vi "Modal Sub-VI.vi"(8 "error in (no error)":errorcluster) -> (0 "error out":errorcluster)   [LabVIEW 2026]
panel:
  out "File Name 1":string caption="File Name"
  in  "Frame Sync Edge for Channel 0":enum16{"Rising", "Falling"}(ring)=enum."Falling"
  in  "Endianness":enum16{"MSB First", "LSB First"}(ring)
  in  "Data Justification":enum16{"Left Justified", "Right Justified"}(ring)
  in  "Channel Count Per Frame":i32=2
  in  "Channel Length":i32=32
  in  "Bit Depth":i32=24
  in  "Channel 0 Offset":i32=1
  in  "Frame Length":i32=64
  in  "Frame Sync Pulse Width":i32=32
  in  "Bit Clock Edge  Sync":enum16{"Rising", "Falling"}(ring)=enum."Falling"
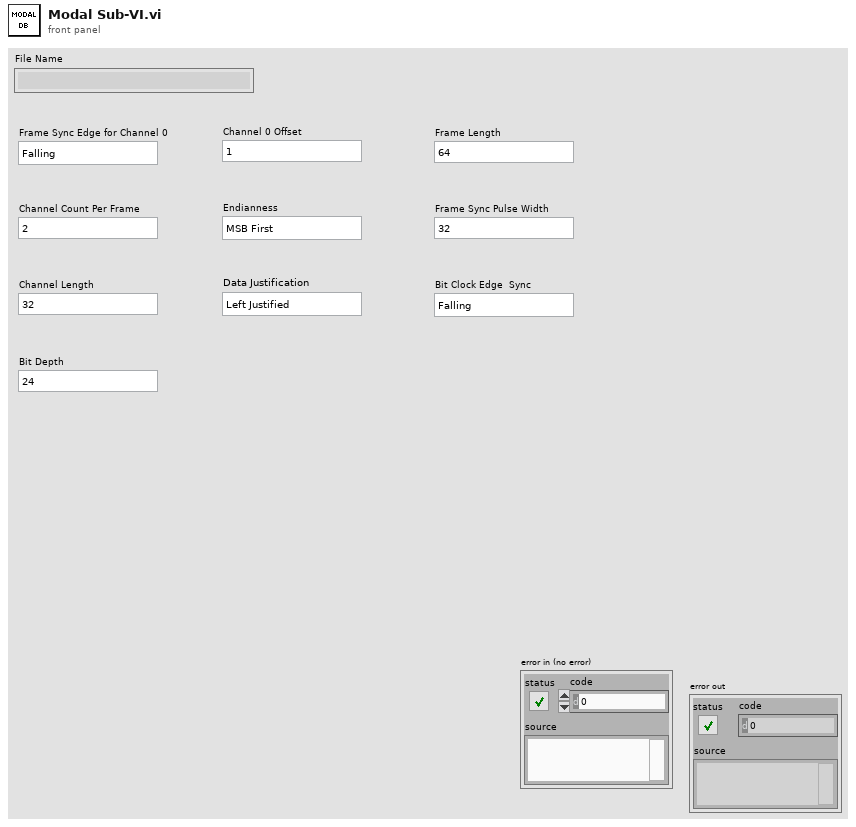
[diagram p1: front panel]
types:
  T1 = enum32{"Invalid", "Standard", "Closed", "Hidden", "Minimized", "Maximized"}
  T2 = cluster{"Configurations":cluster{"Frame_Sync_Edge_for_Channel 0":i32, "Channel_Count_Per_Frame":i32, "Channel_Length":i32, "Bit_Depth":i32, "Channel_0_Offset":i32, "Endianness":i32, "Data_Justification":i32, "Frame_Length":i32, "Frame_Sync_Pulse_Width":i32, "Bit_Clock_Edge_Sync":i32}}
  T3 = enum16{"open", "replace", "create", "open or create", "replace or create", "replace or create with confirmation"}
  T4 = cluster{"Frame_Sync_Edge_for_Channel 0":i32, "Channel_Count_Per_Frame":i32, "Channel_Length":i32, "Bit_Depth":i32, "Channel_0_Offset":i32, "Endianness":i32, "Data_Justification":i32, "Frame_Length":i32, "Frame_Sync_Pulse_Width":i32, "Bit_Clock_Edge_Sync":i32}
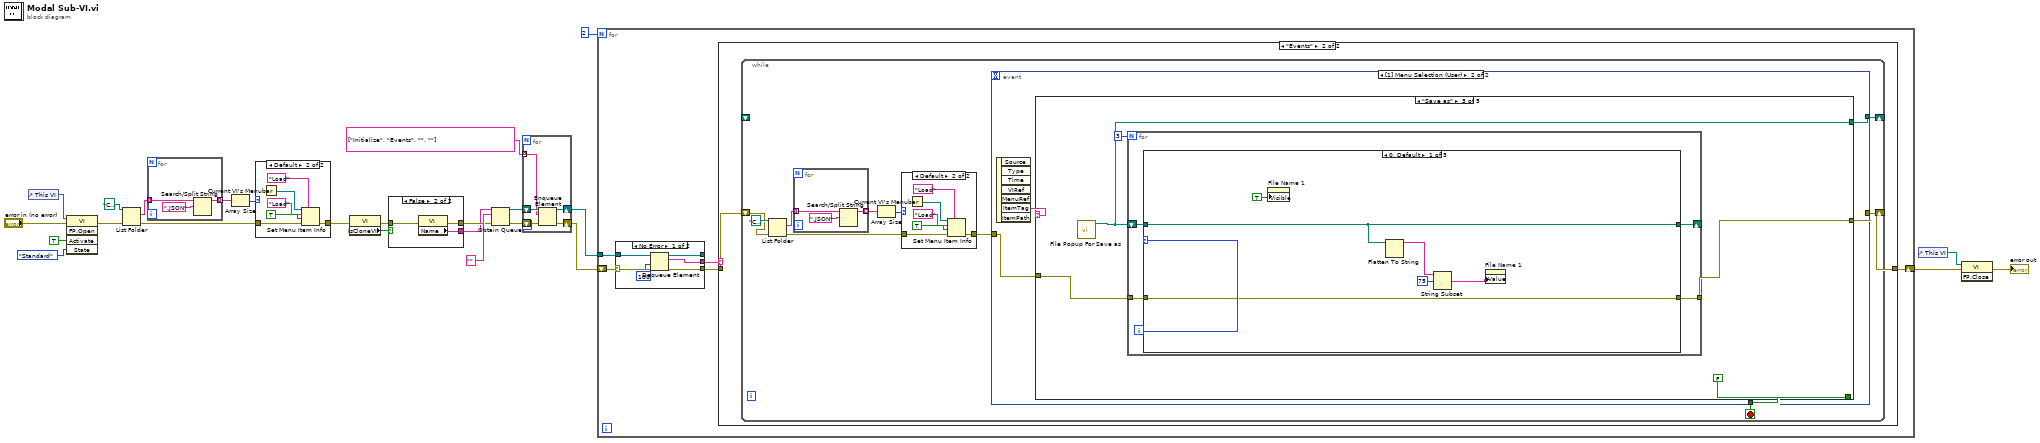
[diagram p0: block diagram]
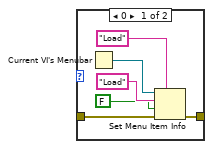
[diagram p2: hidden frame]
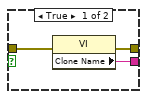
[diagram p3: hidden frame]
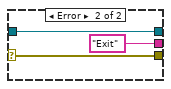
[diagram p4: hidden frame]
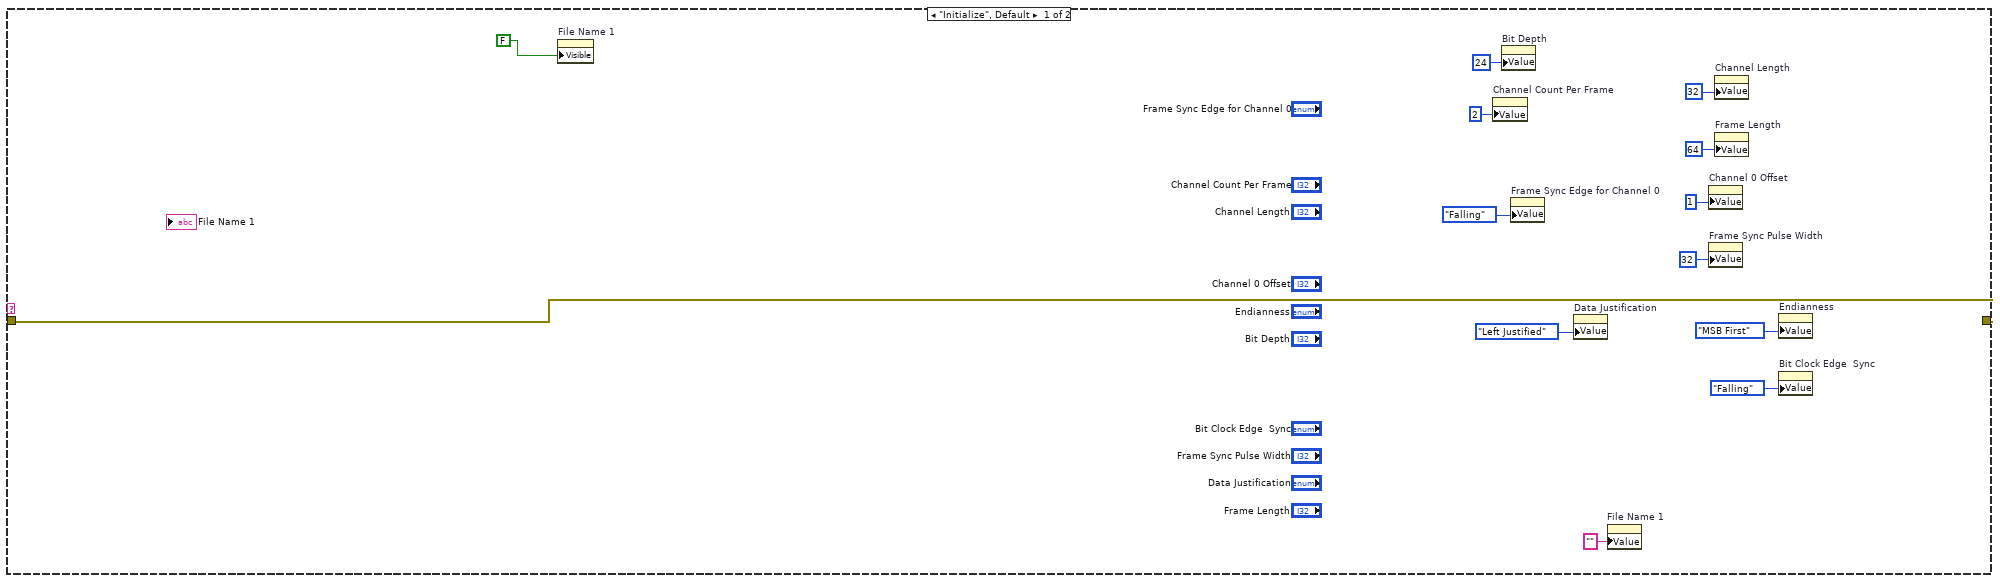
[diagram p5: hidden frame]
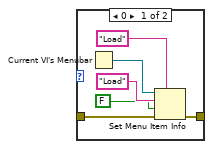
[diagram p6: hidden frame]
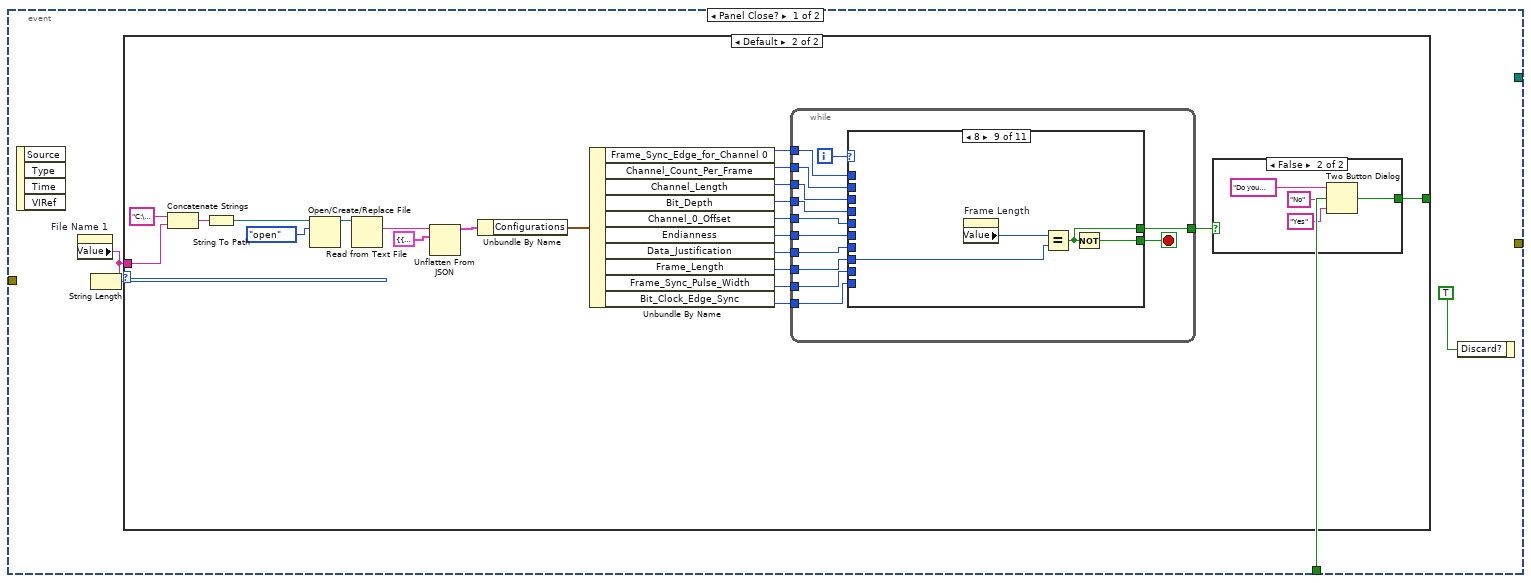
[diagram p7: hidden frame]
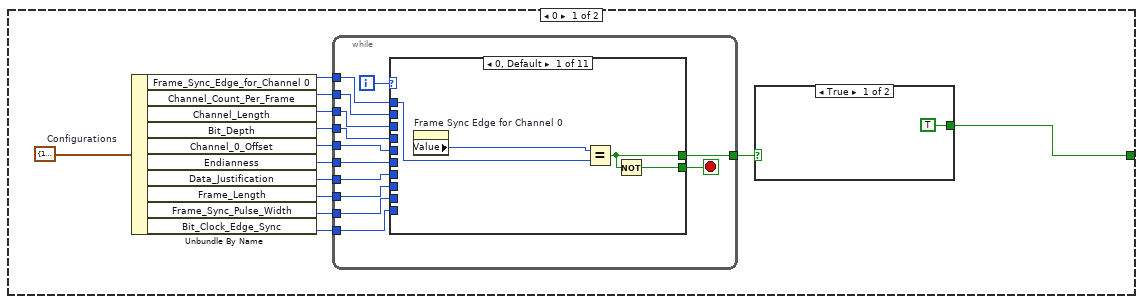
[diagram p8: hidden frame]
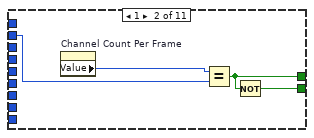
[diagram p9: hidden frame]
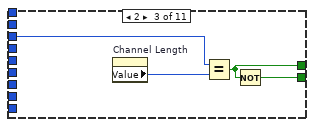
[diagram p10: hidden frame]
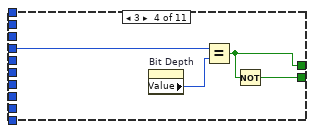
[diagram p11: hidden frame]
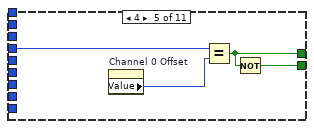
[diagram p12: hidden frame]
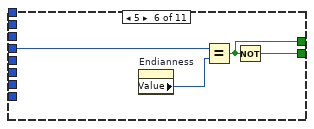
[diagram p13: hidden frame]
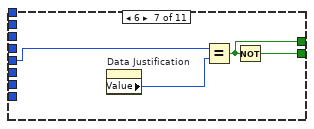
[diagram p14: hidden frame]
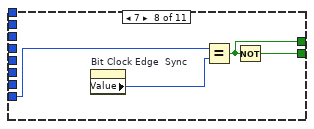
[diagram p15: hidden frame]
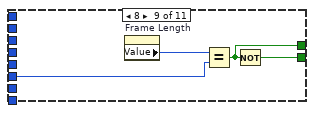
[diagram p16: hidden frame]
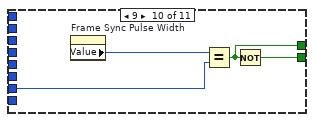
[diagram p17: hidden frame]
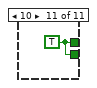
[diagram p18: hidden frame]
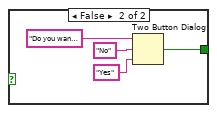
[diagram p19: hidden frame]
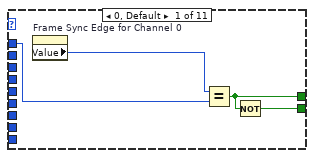
[diagram p20: hidden frame]
diagram:
  n1 = control-ref of="This VI"() -> (w25:refnum<vi>)
  n2 = invoke class="VI" method="FP.Open"(reference=w25, error in="error in (no error)", "Activate"=TRUE ("Activate?"), "State"=T1."Standard") -> (error out=w2:errorcluster)  [unwired: 1 in, 4 out]
  n3 = List Folder(path=path "C:/Users/Public/Documents/National Instruments/Audio/Protocols", error in=w2) -> (filenames=w3:string[], error out=w7:errorcluster)  [unwired: 2 in, 2 out]
  n4 = for {
    tunnel: w3 -> [w27] mode=indexing
    tunnel: [w26] -> w5 mode=indexing
    n5 = Search/Split String(string=w27, search string/char (-)=".JSON") -> (substring before match=w26:string)  [unwired: 1 in, 2 out]
  }
  n6 = Array Size(array=w5) -> (size(s)=w6:i32)
  n7 = case shown="Default" w6 {
    tunnel: w7 -> [w31 w38]
    tunnel: [w30 w37] -> w1
    frame 0 {
      n8 = Current VI's Menubar() -> (w34:refnum<k9>)
      n9 = Set Menu Item Info(7:"Load" ("item tag"), 8:w31, 9:FALSE ("enabled"), 10:"Load" ("item name"), 11:w34) -> (0:w30:errorcluster)  [unwired: 2 in, 1 out]
    }
    frame Default {
      n10 = Current VI's Menubar() -> (w35:refnum<k9>)
      n11 = Set Menu Item Info(7:"Load" ("item tag"), 8:w38, 9:TRUE ("enabled"), 10:"Load" ("item name"), 11:w35) -> (0:w37:errorcluster)  [unwired: 2 in, 1 out]
    }
  }
  n12 = property class="VI"(error in=w1) -> (error out=w14:errorcluster, "IsCloneVI"=w15:bool)  [unwired: 1 in, 1 out]
  n13 = case shown="False" w15 {
    tunnel: [w43 w46] -> w13
    tunnel: [w42 w45] -> w12
    tunnel: w14 -> [w41 w44]
    frame True {
      n14 = property class="VI"(error in=w41) -> (error out=w43:errorcluster, "Clone Name"=w42:string)  [unwired: 1 in, 1 out]
    }
    frame False {
      n15 = property class="VI"(error in=w44) -> (error out=w46:errorcluster, "Name"=w45:string)  [unwired: 1 in, 1 out]
    }
  }
  n16 = Obtain Queue(name (unnamed)=w12, element data type="", error in (no error)=w13) -> (queue out=w16:refnum<queue>, error out=w11:errorcluster)  [unwired: 2 in, 1 out]
  n17 = for {
    shift-right: [w49] -> w9
    shift-left: w16 -> [w51]
    shift-right: [w48] -> w8
    shift-left: w11 -> [w50]
    tunnel: string[] ["Initialize", "Events", "", ""] ("Step sequence") -> [w47] mode=indexing
    n18 = Enqueue Element(queue=w51, element=w47, error in (no error)=w50) -> (queue out=w49:refnum<queue>, error out=w48:errorcluster)  [unwired: 1 in, 1 out]
  }
  n19 = for {
    N: 2 -> [_]
    shift-right: [w52] -> w21
    shift-left: w8 -> [w54]
    tunnel: w9 -> [w56]
    n20 = case shown="No Error" w54 {
      selector: w54 -> [w60 w64]
      tunnel: w56 -> [w62 w63]
      tunnel: [w61 "Exit" ("t")] -> w55
      tunnel: [w59 w64] -> w53
      tunnel: [w57 w63] -> _
      frame No Error {
        n21 = Dequeue Element(queue=w62, timeout in ms (-1)=100, error in (no error)=w60) -> (queue out=w57:refnum<queue>, element=w61:string, error out=w59:errorcluster)  [unwired: 1 out]
      }
      frame Error {
      }
    }
    n22 = case shown="\"Events\"" w55 {
      tunnel: w53 -> [w77 w79]
      tunnel: [w77 w80] -> w52
      frame "Initialize", Default {
        n23 = property on="File Name 1" class="Str"("Visible"=FALSE) -> ()  [unwired: 2 in, 2 out]
        n24 = property on="Channel Count Per Frame" class="DigNum (strict)"("Value"=2 ("Channel Count Per Frame")) -> ()  [unwired: 2 in, 2 out]
        n25 = property on="Bit Depth" class="DigNum (strict)"("Value"=24 ("Bit Depth")) -> ()  [unwired: 2 in, 2 out]
        n26 = property on="Frame Sync Edge for Channel 0" class="Enum (strict)"("Value"=enum16{"Rising", "Falling"}."Falling" ("Frame Sync Edge for Channel 0")) -> ()  [unwired: 2 in, 2 out]
        n27 = property on="Data Justification" class="Enum (strict)"("Value"=enum16{"Left Justified", "Right Justified"}."Left Justified" ("Data Justification")) -> ()  [unwired: 2 in, 2 out]
        n28 = property on="File Name 1" class="Str"("Value"="" ("File Name 1")) -> ()  [unwired: 2 in, 2 out]
        n29 = property on="Channel 0 Offset" class="DigNum (strict)"("Value"=1 ("Channel 0 Offset")) -> ()  [unwired: 2 in, 2 out]
        n30 = property on="Frame Sync Pulse Width" class="DigNum (strict)"("Value"=32 ("Frame Sync Pulse Width")) -> ()  [unwired: 2 in, 2 out]
        n31 = property on="Channel Length" class="DigNum (strict)"("Value"=32 ("Channel Length")) -> ()  [unwired: 2 in, 2 out]
        n32 = property on="Frame Length" class="DigNum (strict)"("Value"=64 ("Frame Length")) -> ()  [unwired: 2 in, 2 out]
        n33 = property on="Endianness" class="Enum (strict)"("Value"=enum16{"MSB First", "LSB First"}."MSB First" ("Endianness")) -> ()  [unwired: 2 in, 2 out]
        n34 = property on="Bit Clock Edge  Sync" class="Enum (strict)"("Value"=enum16{"Rising", "Falling"}."Falling" ("Bit Clock Edge  Sync")) -> ()  [unwired: 2 in, 2 out]
      }
      frame "Events" {
        n35 = while {
          shift-right: [w90] -> w80
          shift-left: w79 -> [w83]
          shift-right: [w81] -> _
          shift-left: _ -> [_]
          stop <- w89 stop-if-true
          n36 = List Folder(path=path "C:/Users/Public/Documents/National Instruments/Audio/Protocols", error in=w83) -> (filenames=w84:string[], error out=w88:errorcluster)  [unwired: 2 in, 2 out]
          n37 = for {
            tunnel: w84 -> [w104] mode=indexing
            tunnel: [w103] -> w86 mode=indexing
            n38 = Search/Split String(string=w104, search string/char (-)=".JSON") -> (substring before match=w103:string)  [unwired: 1 in, 2 out]
          }
          n39 = Array Size(array=w86) -> (size(s)=w87:i32)
          n40 = case shown="Default" w87 {
            tunnel: w88 -> [w93 w100]
            tunnel: [w92 w99] -> w82
            frame 0 {
              n41 = Current VI's Menubar() -> (w96:refnum<k9>)
              n42 = Set Menu Item Info(7:"Load" ("item tag"), 8:w93, 9:FALSE ("enabled"), 10:"Load" ("item name"), 11:w96) -> (0:w92:errorcluster)  [unwired: 2 in, 1 out]
            }
            frame Default {
              n43 = Current VI's Menubar() -> (w97:refnum<k9>)
              n44 = Set Menu Item Info(7:"Load" ("item tag"), 8:w100, 9:TRUE ("enabled"), 10:"Load" ("item name"), 11:w97) -> (0:w99:errorcluster)  [unwired: 2 in, 1 out]
            }
          }
          n45 = event shown="[1] Menu Selection (User)" {
            selector: _ -> [_ _]
            dyn-events: _ -> [_ _]
            timeout: _ -> [_ _]
            tunnel: [_ w267] -> w90
            tunnel: [w107 w265] -> w89
            tunnel: w82 -> [_ w266]
            tunnel: [_ w263] -> w81
            event Panel Close? {
              n46 = event-data() -> ()  [unwired: 1 in, 4 out]
              n47 = property on="File Name 1" class="Str"() -> ("Value"=w106:string)  [unwired: 2 in, 2 out]
              n48 = String Length(string=w106) -> (length=w108:i32)
              n49 = case shown="Default" w108 {
                tunnel: [w111 w186] -> w107
                tunnel: w106 -> [_ w185]
                frame 0 {
                  w122 = T4 {"Frame_Sync_Edge_for_Channel 0"=1, "Channel_Count_Per_Frame"=2, "Channel_Length"=32, "Bit_Depth"=24, "Channel_0_Offset"=1, "Endianness"=0, "Data_Justification"=0, "Frame_Length"=64, "Frame_Sync_Pulse_Width"=32, "Bit_Clock_Edge_Sync"=1}  # Configurations
                  n50 = Unbundle By Name(w122) -> ("Frame_Sync_Edge_for_Channel 0"=w121:i32, "Channel_Count_Per_Frame"=w120:i32, "Channel_Length"=w119:i32, "Bit_Depth"=w118:i32, "Channel_0_Offset"=w117:i32, "Endianness"=w116:i32, "Data_Justification"=w115:i32, "Frame_Length"=w113:i32, "Frame_Sync_Pulse_Width"=w112:i32, "Bit_Clock_Edge_Sync"=w114:i32)
                  n51 = while {
                    tunnel: w121 -> [w135]
                    tunnel: w120 -> [w134]
                    tunnel: w119 -> [w133]
                    tunnel: w118 -> [w132]
                    tunnel: w117 -> [w131]
                    tunnel: w116 -> [w130]
                    tunnel: w115 -> [w129]
                    tunnel: w114 -> [w128]
                    tunnel: w113 -> [w127]
                    tunnel: w112 -> [w126]
                    tunnel: [w125] -> w110
                    i -> [w123]
                    stop <- w124 stop-if-true
                    n52 = case shown="0, Default" w123 {
                      tunnel: w135 -> [w138 _ _ _ _ _ _ _ _ _ _]
                      tunnel: [w137 w141 w145 w149 w153 w157 w161 w165 w169 w173 w176] -> w125
                      tunnel: w134 -> [_ w143 _ _ _ _ _ _ _ _ _]
                      tunnel: w133 -> [_ _ w147 _ _ _ _ _ _ _ _]
                      tunnel: w132 -> [_ _ _ w151 _ _ _ _ _ _ _]
                      tunnel: w131 -> [_ _ _ _ w155 _ _ _ _ _ _]
                      tunnel: w130 -> [_ _ _ _ _ w159 _ _ _ _ _]
                      tunnel: w129 -> [_ _ _ _ _ _ w163 _ _ _ _]
                      tunnel: w128 -> [_ _ _ _ _ _ _ w166 _ _ _]
                      tunnel: w127 -> [_ _ _ _ _ _ _ _ w170 _ _]
                      tunnel: w126 -> [_ _ _ _ _ _ _ _ _ w174 _]
                      tunnel: [w136 w140 w144 w148 w152 w156 w160 w164 w168 w172 w176] -> w124
                      frame 0, Default {
                        n53 = property on="Frame Sync Edge for Channel 0" class="Enum (strict)"() -> ("Value"=w139:enum16{"Rising", "Falling"})  [unwired: 2 in, 2 out]
                        n54 = Equal?(x=w139, y=w138) -> (x = y?=w137:bool)
                        n55 = Not(x=w137) -> (.not. x?=w136:bool)
                      }
                      frame 1 {
                        n56 = property on="Channel Count Per Frame" class="DigNum (strict)"() -> ("Value"=w142:i32)  [unwired: 2 in, 2 out]
                        n57 = Equal?(x=w142, y=w143) -> (x = y?=w141:bool)
                        n58 = Not(x=w141) -> (.not. x?=w140:bool)
                      }
                      frame 2 {
                        n59 = property on="Channel Length" class="DigNum (strict)"() -> ("Value"=w146:i32)  [unwired: 2 in, 2 out]
                        n60 = Equal?(x=w147, y=w146) -> (x = y?=w145:bool)
                        n61 = Not(x=w145) -> (.not. x?=w144:bool)
                      }
                      frame 3 {
                        n62 = property on="Bit Depth" class="DigNum (strict)"() -> ("Value"=w150:i32)  [unwired: 2 in, 2 out]
                        n63 = Equal?(x=w151, y=w150) -> (x = y?=w149:bool)
                        n64 = Not(x=w149) -> (.not. x?=w148:bool)
                      }
                      frame 4 {
                        n65 = property on="Channel 0 Offset" class="DigNum (strict)"() -> ("Value"=w154:i32)  [unwired: 2 in, 2 out]
                        n66 = Equal?(x=w155, y=w154) -> (x = y?=w153:bool)
                        n67 = Not(x=w153) -> (.not. x?=w152:bool)
                      }
                      frame 5 {
                        n68 = property on="Endianness" class="Enum (strict)"() -> ("Value"=w158:enum16{"MSB First", "LSB First"})  [unwired: 2 in, 2 out]
                        n69 = Equal?(x=w159, y=w158) -> (x = y?=w157:bool)
                        n70 = Not(x=w157) -> (.not. x?=w156:bool)
                      }
                      frame 6 {
                        n71 = property on="Data Justification" class="Enum (strict)"() -> ("Value"=w162:enum16{"Left Justified", "Right Justified"})  [unwired: 2 in, 2 out]
                        n72 = Equal?(x=w163, y=w162) -> (x = y?=w161:bool)
                        n73 = Not(x=w161) -> (.not. x?=w160:bool)
                      }
                      frame 7 {
                        n74 = property on="Bit Clock Edge  Sync" class="Enum (strict)"() -> ("Value"=w167:enum16{"Rising", "Falling"})  [unwired: 2 in, 2 out]
                        n75 = Equal?(x=w166, y=w167) -> (x = y?=w165:bool)
                        n76 = Not(x=w165) -> (.not. x?=w164:bool)
                      }
                      frame 8 {
                        n77 = property on="Frame Length" class="DigNum (strict)"() -> ("Value"=w171:i32)  [unwired: 2 in, 2 out]
                        n78 = Equal?(x=w171, y=w170) -> (x = y?=w169:bool)
                        n79 = Not(x=w169) -> (.not. x?=w168:bool)
                      }
                      frame 9 {
                        n80 = property on="Frame Sync Pulse Width" class="DigNum (strict)"() -> ("Value"=w175:i32)  [unwired: 2 in, 2 out]
                        n81 = Equal?(x=w175, y=w174) -> (x = y?=w173:bool)
                        n82 = Not(x=w173) -> (.not. x?=w172:bool)
                      }
                      frame 10 {
                        w176 = TRUE
                      }
                    }
                  }
                  n83 = case shown="True" w110 {
                    tunnel: [TRUE ("T button?") w181] -> w111
                    frame True {
                    }
                    frame False {
                      n84 = Two Button Dialog(message="Do you want to save the changes in configurations?", 1:"Yes" ("F button name (\"Cancel\")"), 2:"No" ("T button name (\"OK\")")) -> (T button?=w181:bool)
                    }
                  }
                }
                frame Default {
                  n85 = Concatenate Strings("C:\\Users\\Public\\Documents\\National Instruments\\Audio\\Protocols\\" ("string"), w185) -> (w183:string)
                  n86 = String To Path(string=w183) -> (path=w182:path)
                  n87 = Open/Create/Replace File(file path (use dialog)=w182, operation (0:open)=T3."open") -> (refnum out=w202:refnum<file>)  [unwired: 4 in, 2 out]
                  n88 = Read from Text File(file (use dialog)=w202) -> (text=w203:string)  [unwired: 3 in, 3 out]
                  n89 = Unflatten From JSON(JSON string=w203, type and defaults=T2 {"Configurations"={"Frame_Sync_Edge_for_Channel 0"=1, "Channel_Count_Per_Frame"=2, "Channel_Length"=32, "Bit_Depth"=24, "Channel_0_Offset"=1, "Endianness"=0, "Data_Justification"=0, "Frame_Length"=64, "Frame_Sync_Pulse_Width"=32, "Bit_Clock_Edge_Sync"=0}}) -> (value=w201:T2)  [unwired: 5 in, 1 out]
                  n90 = Unbundle By Name(w201) -> ("Configurations"=w187:T4)
                  n91 = Unbundle By Name(w187) -> ("Frame_Sync_Edge_for_Channel 0"=w188:i32, "Channel_Count_Per_Frame"=w189:i32, "Channel_Length"=w190:i32, "Bit_Depth"=w191:i32, "Channel_0_Offset"=w192:i32, "Endianness"=w193:i32, "Data_Justification"=w194:i32, "Frame_Length"=w196:i32, "Frame_Sync_Pulse_Width"=w197:i32, "Bit_Clock_Edge_Sync"=w195:i32)
                  n92 = while {
                    tunnel: [w206] -> w198
                    tunnel: w197 -> [w216]
                    tunnel: w196 -> [w215]
                    tunnel: w195 -> [w214]
                    tunnel: w194 -> [w213]
                    tunnel: w193 -> [w212]
                    tunnel: w192 -> [w211]
                    tunnel: w191 -> [w210]
                    tunnel: w190 -> [w209]
                    tunnel: w189 -> [w208]
                    tunnel: w188 -> [w207]
                    i -> [w205]
                    stop <- w204 stop-if-true
                    n93 = case shown="8" w205 {
                      tunnel: w207 -> [w220 _ _ _ _ _ _ _ _ _ _]
                      tunnel: [w218 w222 w226 w230 w234 w238 w242 w246 w250 w253 w257] -> w206
                      tunnel: w208 -> [_ w224 _ _ _ _ _ _ _ _ _]
                      tunnel: w209 -> [_ _ w228 _ _ _ _ _ _ _ _]
                      tunnel: w210 -> [_ _ _ w232 _ _ _ _ _ _ _]
                      tunnel: w211 -> [_ _ _ _ w236 _ _ _ _ _ _]
                      tunnel: w212 -> [_ _ _ _ _ w240 _ _ _ _ _]
                      tunnel: w213 -> [_ _ _ _ _ _ w244 _ _ _ _]
                      tunnel: w214 -> [_ _ _ _ _ _ _ w248 _ _ _]
                      tunnel: w215 -> [_ _ _ _ _ _ _ _ w252 _ _]
                      tunnel: w216 -> [_ _ _ _ _ _ _ _ _ w256 _]
                      tunnel: [w217 w221 w225 w229 w233 w237 w241 w245 w249 w254 w257] -> w204
                      frame 0, Default {
                        n94 = property on="Frame Sync Edge for Channel 0" class="Enum (strict)"() -> ("Value"=w219:enum16{"Rising", "Falling"})  [unwired: 2 in, 2 out]
                        n95 = Equal?(x=w219, y=w220) -> (x = y?=w218:bool)
                        n96 = Not(x=w218) -> (.not. x?=w217:bool)
                      }
                      frame 1 {
                        n97 = property on="Channel Count Per Frame" class="DigNum (strict)"() -> ("Value"=w223:i32)  [unwired: 2 in, 2 out]
                        n98 = Equal?(x=w223, y=w224) -> (x = y?=w222:bool)
                        n99 = Not(x=w222) -> (.not. x?=w221:bool)
                      }
                      frame 2 {
                        n100 = property on="Channel Length" class="DigNum (strict)"() -> ("Value"=w227:i32)  [unwired: 2 in, 2 out]
                        n101 = Equal?(x=w228, y=w227) -> (x = y?=w226:bool)
                        n102 = Not(x=w226) -> (.not. x?=w225:bool)
                      }
                      frame 3 {
                        n103 = property on="Bit Depth" class="DigNum (strict)"() -> ("Value"=w231:i32)  [unwired: 2 in, 2 out]
                        n104 = Equal?(x=w232, y=w231) -> (x = y?=w230:bool)
                        n105 = Not(x=w230) -> (.not. x?=w229:bool)
                      }
                      frame 4 {
                        n106 = property on="Channel 0 Offset" class="DigNum (strict)"() -> ("Value"=w235:i32)  [unwired: 2 in, 2 out]
                        n107 = Equal?(x=w236, y=w235) -> (x = y?=w234:bool)
                        n108 = Not(x=w234) -> (.not. x?=w233:bool)
                      }
                      frame 5 {
                        n109 = property on="Endianness" class="Enum (strict)"() -> ("Value"=w239:enum16{"MSB First", "LSB First"})  [unwired: 2 in, 2 out]
                        n110 = Equal?(x=w240, y=w239) -> (x = y?=w238:bool)
                        n111 = Not(x=w238) -> (.not. x?=w237:bool)
                      }
                      frame 6 {
                        n112 = property on="Data Justification" class="Enum (strict)"() -> ("Value"=w243:enum16{"Left Justified", "Right Justified"})  [unwired: 2 in, 2 out]
                        n113 = Equal?(x=w244, y=w243) -> (x = y?=w242:bool)
                        n114 = Not(x=w242) -> (.not. x?=w241:bool)
                      }
                      frame 7 {
                        n115 = property on="Bit Clock Edge  Sync" class="Enum (strict)"() -> ("Value"=w247:enum16{"Rising", "Falling"})  [unwired: 2 in, 2 out]
                        n116 = Equal?(x=w248, y=w247) -> (x = y?=w246:bool)
                        n117 = Not(x=w246) -> (.not. x?=w245:bool)
                      }
                      frame 8 {
                        n118 = property on="Frame Length" class="DigNum (strict)"() -> ("Value"=w251:i32)  [unwired: 2 in, 2 out]
                        n119 = Equal?(x=w251, y=w252) -> (x = y?=w250:bool)
                        n120 = Not(x=w250) -> (.not. x?=w249:bool)
                      }
                      frame 9 {
                        n121 = property on="Frame Sync Pulse Width" class="DigNum (strict)"() -> ("Value"=w255:i32)  [unwired: 2 in, 2 out]
                        n122 = Equal?(x=w255, y=w256) -> (x = y?=w253:bool)
                        n123 = Not(x=w253) -> (.not. x?=w254:bool)
                      }
                      frame 10 {
                        w257 = TRUE
                      }
                    }
                  }
                  n124 = case shown="False" w198 {
                    tunnel: [TRUE ("T button?") w262] -> w186
                    frame True {
                    }
                    frame False {
                      n125 = Two Button Dialog(message="Do you want to save changes in file?", 1:"Yes" ("F button name (\"Cancel\")"), 2:"No" ("T button name (\"OK\")")) -> (T button?=w262:bool)
                    }
                  }
                }
              }
              n126 = event-data("Discard?"=TRUE) -> ()  [unwired: 1 in, 1 out]
            }
            event Menu Selection (User) {
              n127 = event-data() -> ("ItemTag"=w264:string)  [unwired: 1 in, 6 out]
              n128 = case shown="\"Save as\"" w264 {
                tunnel: [w268 w272 w333 w421 w422] -> w267
                tunnel: w266 -> [w268 w274 w334 w394 w423]
                tunnel: [FALSE FALSE FALSE FALSE w424] -> w265
                tunnel: [_ w270 w331 w392 _] -> w263
                frame "File", Default {
                }
                frame "Save" {
                  n129 = for {
                    N: 3 -> [_]
                    tunnel: w274 -> [w279]
                    tunnel: [w275] -> w272
                    shift-right: [w277] -> w270
                    shift-left: _ -> [w276]
                    i -> [w278]
                    n130 = case shown="0, Default" w278 {
                      tunnel: w279 -> [w281 w288 w319]
                      tunnel: [w280 w287 w310] -> w277
                      tunnel: w276 -> [_ w287 w310]
                      tunnel: [w281 w286 w320] -> w275
                      frame 0, Default {
                        n131 = property on="File Name 1" class="Str"("Visible"=TRUE) -> ()  [unwired: 2 in, 2 out]
                        n132 = call "File Popup For Save.vi"() -> ("selected path"=w280:path)  [unwired: 9 in, 2 out]
                        n133 = Flatten To String(anything=w280) -> (data string=w284:string)  [unwired: 3 in, 2 out]
                        n134 = String Subset(string=w284, offset (0)=75) -> (substring=w283:string)  [unwired: 1 in]
                        n135 = property on="File Name 1" class="Str"("Value"=w283) -> ()  [unwired: 2 in, 2 out]
                      }
                      frame 1 {
                        w289 = T4 {"Frame_Sync_Edge_for_Channel 0"=1, "Channel_Count_Per_Frame"=2, "Channel_Length"=32, "Bit_Depth"=24, "Channel_0_Offset"=1, "Endianness"=0, "Data_Justification"=0, "Frame_Length"=0, "Frame_Sync_Pulse_Width"=0, "Bit_Clock_Edge_Sync"=0}  # Configurations
                        n136 = property on="Endianness" class="Enum (strict)"() -> ("Value"=w297:enum16{"MSB First", "LSB First"})  [unwired: 2 in, 2 out]
                        n137 = property on="Frame Length" class="DigNum (strict)"() -> ("Value"=w299:i32)  [unwired: 2 in, 2 out]
                        n138 = property on="Frame Sync Pulse Width" class="DigNum (strict)"() -> ("Value"=w300:i32)  [unwired: 2 in, 2 out]
                        n139 = property on="Bit Clock Edge  Sync" class="Enum (strict)"() -> ("Value"=w301:enum16{"Rising", "Falling"})  [unwired: 2 in, 2 out]
                        n140 = property on="Channel 0 Offset" class="DigNum (strict)"() -> ("Value"=w296:i32)  [unwired: 2 in, 2 out]
                        n141 = property on="Channel Count Per Frame" class="DigNum (strict)"() -> ("Value"=w294:i32)  [unwired: 2 in, 2 out]
                        n142 = property on="Channel Length" class="DigNum (strict)"() -> ("Value"=w293:i32)  [unwired: 2 in, 2 out]
                        n143 = property on="Bit Depth" class="DigNum (strict)"() -> ("Value"=w292:i32)  [unwired: 2 in, 2 out]
                        n144 = property on="Frame Sync Edge for Channel 0" class="Enum (strict)"() -> ("Value"=w295:enum16{"Rising", "Falling"})  [unwired: 2 in, 2 out]
                        n145 = property on="Data Justification" class="Enum (strict)"() -> ("Value"=w298:enum16{"Left Justified", "Right Justified"})  [unwired: 2 in, 2 out]
                        n146 = Bundle By Name(cluster=w289, "Frame_Sync_Edge_for_Channel 0"=w295, "Channel_Count_Per_Frame"=w294, "Channel_Length"=w293, "Bit_Depth"=w292, "Channel_0_Offset"=w296, "Endianness"=w297, "Data_Justification"=w298, "Frame_Length"=w299, "Frame_Sync_Pulse_Width"=w300, "Bit_Clock_Edge_Sync"=w301) -> (w309:T4)
                        n147 = Bundle By Name(cluster=T2 {"Configurations"={"Frame_Sync_Edge_for_Channel 0"=1, "Channel_Count_Per_Frame"=2, "Channel_Length"=32, "Bit_Depth"=24, "Channel_0_Offset"=1, "Endianness"=0, "Data_Justification"=0, "Frame_Length"=0, "Frame_Sync_Pulse_Width"=0, "Bit_Clock_Edge_Sync"=0}}, "Configurations"=w309) -> (w308:T2)
                        n148 = Open/Create/Replace File(file path (use dialog)=w287, error in=w288, operation (0:open)=T3."replace or create") -> (refnum out=w306:refnum<file>, error out=w307:errorcluster)  [unwired: 3 in, 1 out]
                        n149 = Flatten To JSON(anything=w308, error in (no error)=w307) -> (JSON string=w303:string, 11:w304:errorcluster)  [unwired: 1 in]
                        n150 = Write to Text File(file (use dialog)=w306, text=w303, error in=w304) -> (refnum out=w302:refnum<file>, error out=w305:errorcluster)  [unwired: 1 in, 1 out]
                        n151 = Close File(refnum=w302, error in=w305) -> (error out=w286:errorcluster)  [unwired: 1 out]
                      }
                      frame 2 {
                        n152 = Open/Create/Replace File(file path (use dialog)=w310, error in=w319, operation (0:open)=T3."open") -> (refnum out=w328:refnum<file>, error out=w326:errorcluster)  [unwired: 3 in, 1 out]
                        n153 = Read from Text File(file (use dialog)=w328, error in=w326) -> (text=w329:string, error out=w327:errorcluster)  [unwired: 2 in, 2 out]
                        n154 = Unflatten From JSON(JSON string=w329, type and defaults=T2 {"Configurations"={"Frame_Sync_Edge_for_Channel 0"=1, "Channel_Count_Per_Frame"=2, "Channel_Length"=32, "Bit_Depth"=24, "Channel_0_Offset"=1, "Endianness"=0, "Data_Justification"=0, "Frame_Length"=64, "Frame_Sync_Pulse_Width"=32, "Bit_Clock_Edge_Sync"=0}}, error in (no error)=w327) -> (value=w325:T2, error out=w320:errorcluster)  [unwired: 4 in]
                        n155 = Unbundle By Name(w325) -> ("Configurations"=w330:T4)
                        n156 = Unbundle By Name(w330) -> ("Frame_Sync_Edge_for_Channel 0"=w311:i32, "Channel_Count_Per_Frame"=w322:i32, "Channel_Length"=w321:i32, "Bit_Depth"=w318:i32, "Channel_0_Offset"=w317:i32, "Endianness"=w316:i32, "Data_Justification"=w315:i32, "Frame_Length"=w314:i32, "Frame_Sync_Pulse_Width"=w313:i32, "Bit_Clock_Edge_Sync"=w312:i32)
                        n157 = property on="Frame Sync Edge for Channel 0" class="Enum (strict)"("Value"=w311) -> ()  [unwired: 2 in, 2 out]
                        n158 = property on="Channel Count Per Frame" class="DigNum (strict)"("Value"=w322) -> ()  [unwired: 2 in, 2 out]
                        n159 = property on="Channel Length" class="DigNum (strict)"("Value"=w321) -> ()  [unwired: 2 in, 2 out]
                        n160 = property on="Bit Depth" class="DigNum (strict)"("Value"=w318) -> ()  [unwired: 2 in, 2 out]
                        n161 = property on="Channel 0 Offset" class="DigNum (strict)"("Value"=w317) -> ()  [unwired: 2 in, 2 out]
                        n162 = property on="Endianness" class="Enum (strict)"("Value"=w316) -> ()  [unwired: 2 in, 2 out]
                        n163 = property on="Data Justification" class="Enum (strict)"("Value"=w315) -> ()  [unwired: 2 in, 2 out]
                        n164 = property on="Frame Length" class="DigNum (strict)"("Value"=w314) -> ()  [unwired: 2 in, 2 out]
                        n165 = property on="Frame Sync Pulse Width" class="DigNum (strict)"("Value"=w313) -> ()  [unwired: 2 in, 2 out]
                        n166 = property on="Bit Clock Edge  Sync" class="Enum (strict)"("Value"=w312) -> ()  [unwired: 2 in, 2 out]
                      }
                    }
                  }
                }
                frame "Save as" {
                  n167 = call "File Popup For Save as.vi"() -> ("selected path"=w331:path)  [unwired: 8 in, 3 out]
                  n168 = for {
                    N: 3 -> [_]
                    tunnel: w334 -> [w340]
                    tunnel: [w336] -> w333
                    shift-right: [w338] -> _
                    shift-left: w331 -> [w337]
                    i -> [w339]
                    n169 = case shown="0, Default" w339 {
                      tunnel: w340 -> [w343 w359 w382]
                      tunnel: [w344 w347 _] -> w338
                      tunnel: w337 -> [w344 w347 w383]
                      tunnel: [w343 w358 w376] -> w336
                      frame 0, Default {
                        n170 = property on="File Name 1" class="Str"("Visible"=TRUE) -> ()  [unwired: 2 in, 2 out]
                        n171 = Flatten To String(anything=w344) -> (data string=w346:string)  [unwired: 3 in, 2 out]
                        n172 = String Subset(string=w346, offset (0)=75) -> (substring=w342:string)  [unwired: 1 in]
                        n173 = property on="File Name 1" class="Str"("Value"=w342) -> ()  [unwired: 2 in, 2 out]
                      }
                      frame 1 {
                        w360 = T4 {"Frame_Sync_Edge_for_Channel 0"=1, "Channel_Count_Per_Frame"=2, "Channel_Length"=32, "Bit_Depth"=24, "Channel_0_Offset"=1, "Endianness"=0, "Data_Justification"=0, "Frame_Length"=0, "Frame_Sync_Pulse_Width"=0, "Bit_Clock_Edge_Sync"=0}  # Configurations
                        n174 = property on="Frame Sync Edge for Channel 0" class="Enum (strict)"() -> ("Value"=w357:enum16{"Rising", "Falling"})  [unwired: 2 in, 2 out]
                        n175 = property on="Channel Count Per Frame" class="DigNum (strict)"() -> ("Value"=w356:i32)  [unwired: 2 in, 2 out]
                        n176 = property on="Channel Length" class="DigNum (strict)"() -> ("Value"=w355:i32)  [unwired: 2 in, 2 out]
                        n177 = property on="Bit Depth" class="DigNum (strict)"() -> ("Value"=w354:i32)  [unwired: 2 in, 2 out]
                        n178 = property on="Channel 0 Offset" class="DigNum (strict)"() -> ("Value"=w353:i32)  [unwired: 2 in, 2 out]
                        n179 = property on="Endianness" class="Enum (strict)"() -> ("Value"=w352:enum16{"MSB First", "LSB First"})  [unwired: 2 in, 2 out]
                        n180 = property on="Data Justification" class="Enum (strict)"() -> ("Value"=w351:enum16{"Left Justified", "Right Justified"})  [unwired: 2 in, 2 out]
                        n181 = property on="Frame Length" class="DigNum (strict)"() -> ("Value"=w350:i32)  [unwired: 2 in, 2 out]
                        n182 = property on="Frame Sync Pulse Width" class="DigNum (strict)"() -> ("Value"=w349:i32)  [unwired: 2 in, 2 out]
                        n183 = property on="Bit Clock Edge  Sync" class="Enum (strict)"() -> ("Value"=w348:enum16{"Rising", "Falling"})  [unwired: 2 in, 2 out]
                        n184 = Bundle By Name(cluster=w360, "Frame_Sync_Edge_for_Channel 0"=w357, "Channel_Count_Per_Frame"=w356, "Channel_Length"=w355, "Bit_Depth"=w354, "Channel_0_Offset"=w353, "Endianness"=w352, "Data_Justification"=w351, "Frame_Length"=w350, "Frame_Sync_Pulse_Width"=w349, "Bit_Clock_Edge_Sync"=w348) -> (w370:T4)
                        n185 = Bundle By Name(cluster=T2 {"Configurations"={"Frame_Sync_Edge_for_Channel 0"=1, "Channel_Count_Per_Frame"=2, "Channel_Length"=32, "Bit_Depth"=24, "Channel_0_Offset"=1, "Endianness"=0, "Data_Justification"=0, "Frame_Length"=0, "Frame_Sync_Pulse_Width"=0, "Bit_Clock_Edge_Sync"=0}}, "Configurations"=w370) -> (w369:T2)
                        n186 = Open/Create/Replace File(file path (use dialog)=w347, error in=w359, operation (0:open)=T3."replace or create") -> (refnum out=w367:refnum<file>, error out=w368:errorcluster)  [unwired: 3 in, 1 out]
                        n187 = Flatten To JSON(anything=w369, error in (no error)=w368) -> (JSON string=w364:string, 11:w365:errorcluster)  [unwired: 1 in]
                        n188 = Write to Text File(file (use dialog)=w367, text=w364, error in=w365) -> (refnum out=w363:refnum<file>, error out=w366:errorcluster)  [unwired: 1 in, 1 out]
                        n189 = Close File(refnum=w363, error in=w366) -> (error out=w358:errorcluster)  [unwired: 1 out]
                      }
                      frame 2 {
                        n190 = Open/Create/Replace File(file path (use dialog)=w383, error in=w382, operation (0:open)=T3."open") -> (refnum out=w389:refnum<file>, error out=w387:errorcluster)  [unwired: 3 in, 1 out]
                        n191 = Read from Text File(file (use dialog)=w389, error in=w387) -> (text=w390:string, error out=w388:errorcluster)  [unwired: 2 in, 2 out]
                        n192 = Unflatten From JSON(JSON string=w390, type and defaults=T2 {"Configurations"={"Frame_Sync_Edge_for_Channel 0"=1, "Channel_Count_Per_Frame"=2, "Channel_Length"=32, "Bit_Depth"=24, "Channel_0_Offset"=1, "Endianness"=0, "Data_Justification"=0, "Frame_Length"=64, "Frame_Sync_Pulse_Width"=32, "Bit_Clock_Edge_Sync"=0}}, error in (no error)=w388) -> (value=w386:T2, error out=w376:errorcluster)  [unwired: 4 in]
                        n193 = Unbundle By Name(w386) -> ("Configurations"=w391:T4)
                        n194 = Unbundle By Name(w391) -> ("Frame_Sync_Edge_for_Channel 0"=w381:i32, "Channel_Count_Per_Frame"=w380:i32, "Channel_Length"=w379:i32, "Bit_Depth"=w378:i32, "Channel_0_Offset"=w377:i32, "Endianness"=w375:i32, "Data_Justification"=w374:i32, "Frame_Length"=w373:i32, "Frame_Sync_Pulse_Width"=w372:i32, "Bit_Clock_Edge_Sync"=w371:i32)
                        n195 = property on="Frame Sync Edge for Channel 0" class="Enum (strict)"("Value"=w381) -> ()  [unwired: 2 in, 2 out]
                        n196 = property on="Channel Count Per Frame" class="DigNum (strict)"("Value"=w380) -> ()  [unwired: 2 in, 2 out]
                        n197 = property on="Channel Length" class="DigNum (strict)"("Value"=w379) -> ()  [unwired: 2 in, 2 out]
                        n198 = property on="Bit Depth" class="DigNum (strict)"("Value"=w378) -> ()  [unwired: 2 in, 2 out]
                        n199 = property on="Channel 0 Offset" class="DigNum (strict)"(error in=w376, "Value"=w377) -> ()  [unwired: 1 in, 2 out]
                        n200 = property on="Endianness" class="Enum (strict)"("Value"=w375) -> ()  [unwired: 2 in, 2 out]
                        n201 = property on="Data Justification" class="Enum (strict)"("Value"=w374) -> ()  [unwired: 2 in, 2 out]
                        n202 = property on="Frame Length" class="DigNum (strict)"("Value"=w373) -> ()  [unwired: 2 in, 2 out]
                        n203 = property on="Frame Sync Pulse Width" class="DigNum (strict)"("Value"=w372) -> ()  [unwired: 2 in, 2 out]
                        n204 = property on="Bit Clock Edge  Sync" class="Enum (strict)"("Value"=w371) -> ()  [unwired: 2 in, 2 out]
                      }
                    }
                  }
                }
                frame "Load" {
                  n205 = call "File Popup For Load.vi"("error in (no error)"=w394) -> ("error out"=w393:errorcluster, "selected path"=w392:path)  [unwired: 8 in, 1 out]
                  n206 = Flatten To String(anything=w392, error in (no error)=w393) -> (data string=w419:string, error out=w403:errorcluster)  [unwired: 2 in, 1 out]
                  n207 = String Subset(string=w419, offset (0)=75) -> (substring=w417:string)  [unwired: 1 in]
                  n208 = property on="File Name 1" class="Str"(error in=w403, "Value"=w417) -> (error out=w402:errorcluster)  [unwired: 1 in, 1 out]
                  n209 = property on="File Name 1" class="Str"(error in=w402, "Visible"=TRUE) -> (error out=w401:errorcluster)  [unwired: 1 in, 1 out]
                  n210 = Open/Create/Replace File(file path (use dialog)=w392, error in=w401, operation (0:open)=T3."open") -> (refnum out=w412:refnum<file>, error out=w414:errorcluster)  [unwired: 3 in, 1 out]
                  n211 = Read from Text File(file (use dialog)=w412, error in=w414) -> (text=w411:string, error out=w413:errorcluster)  [unwired: 2 in, 2 out]
                  n212 = Unflatten From JSON(JSON string=w411, type and defaults=T2 {"Configurations"={"Frame_Sync_Edge_for_Channel 0"=1, "Channel_Count_Per_Frame"=2, "Channel_Length"=32, "Bit_Depth"=24, "Channel_0_Offset"=1, "Endianness"=0, "Data_Justification"=0, "Frame_Length"=64, "Frame_Sync_Pulse_Width"=32, "Bit_Clock_Edge_Sync"=0}}, error in (no error)=w413) -> (value=w416:T2, error out=w421:errorcluster)  [unwired: 4 in]
                  n213 = Unbundle By Name(w416) -> ("Configurations"=w409:T4)
                  n214 = Unbundle By Name(w409) -> ("Frame_Sync_Edge_for_Channel 0"=w408:i32, "Channel_Count_Per_Frame"=w397:i32, "Channel_Length"=w399:i32, "Bit_Depth"=w398:i32, "Channel_0_Offset"=w396:i32, "Endianness"=w407:i32, "Data_Justification"=w406:i32, "Frame_Length"=w395:i32, "Frame_Sync_Pulse_Width"=w405:i32, "Bit_Clock_Edge_Sync"=w404:i32)
                  n215 = property on="Frame Sync Edge for Channel 0" class="Enum (strict)"("Value"=w408) -> ()  [unwired: 2 in, 2 out]
                  n216 = property on="Channel Count Per Frame" class="DigNum (strict)"("Value"=w397) -> ()  [unwired: 2 in, 2 out]
                  n217 = property on="Channel Length" class="DigNum (strict)"("Value"=w399) -> ()  [unwired: 2 in, 2 out]
                  n218 = property on="Bit Depth" class="DigNum (strict)"("Value"=w398) -> ()  [unwired: 2 in, 2 out]
                  n219 = property on="Channel 0 Offset" class="DigNum (strict)"("Value"=w396) -> ()  [unwired: 2 in, 2 out]
                  n220 = property on="Endianness" class="Enum (strict)"("Value"=w407) -> ()  [unwired: 2 in, 2 out]
                  n221 = property on="Data Justification" class="Enum (strict)"("Value"=w406) -> ()  [unwired: 2 in, 2 out]
                  n222 = property on="Frame Length" class="DigNum (strict)"("Value"=w395) -> ()  [unwired: 2 in, 2 out]
                  n223 = property on="Frame Sync Pulse Width" class="DigNum (strict)"("Value"=w405) -> ()  [unwired: 2 in, 2 out]
                  n224 = property on="Bit Clock Edge  Sync" class="Enum (strict)"("Value"=w404) -> ()  [unwired: 2 in, 2 out]
                }
                frame "Exit" {
                  n225 = property on="File Name 1" class="Str"() -> ("Value"=w425:string)  [unwired: 2 in, 2 out]
                  n226 = String Length(string=w425) -> (length=w426:i32)
                  n227 = case shown="Default" w426 {
                    tunnel: [w429 w505] -> w424
                    tunnel: w425 -> [_ w504]
                    tunnel: w423 -> [w427 w500]
                    tunnel: [w427 w500] -> w422
                    frame 0 {
                      w440 = T4 {"Frame_Sync_Edge_for_Channel 0"=1, "Channel_Count_Per_Frame"=2, "Channel_Length"=32, "Bit_Depth"=24, "Channel_0_Offset"=1, "Endianness"=0, "Data_Justification"=0, "Frame_Length"=64, "Frame_Sync_Pulse_Width"=32, "Bit_Clock_Edge_Sync"=1}  # Configurations
                      n228 = Unbundle By Name(w440) -> ("Frame_Sync_Edge_for_Channel 0"=w439:i32, "Channel_Count_Per_Frame"=w438:i32, "Channel_Length"=w437:i32, "Bit_Depth"=w436:i32, "Channel_0_Offset"=w435:i32, "Endianness"=w434:i32, "Data_Justification"=w433:i32, "Frame_Length"=w431:i32, "Frame_Sync_Pulse_Width"=w430:i32, "Bit_Clock_Edge_Sync"=w432:i32)
                      n229 = while {
                        tunnel: w439 -> [w453]
                        tunnel: w438 -> [w452]
                        tunnel: w437 -> [w451]
                        tunnel: w436 -> [w450]
                        tunnel: w435 -> [w449]
                        tunnel: w434 -> [w448]
                        tunnel: w433 -> [w447]
                        tunnel: w432 -> [w446]
                        tunnel: w431 -> [w445]
                        tunnel: w430 -> [w444]
                        tunnel: [w443] -> w428
                        i -> [w441]
                        stop <- w442 stop-if-true
                        n230 = case shown="9" w441 {
                          tunnel: w453 -> [w456 _ _ _ _ _ _ _ _ _ _]
                          tunnel: [w455 w459 w463 w467 w471 w475 w479 w483 w487 w491 w494] -> w443
                          tunnel: w452 -> [_ w461 _ _ _ _ _ _ _ _ _]
                          tunnel: w451 -> [_ _ w465 _ _ _ _ _ _ _ _]
                          tunnel: w450 -> [_ _ _ w469 _ _ _ _ _ _ _]
                          tunnel: w449 -> [_ _ _ _ w473 _ _ _ _ _ _]
                          tunnel: w448 -> [_ _ _ _ _ w477 _ _ _ _ _]
                          tunnel: w447 -> [_ _ _ _ _ _ w481 _ _ _ _]
                          tunnel: w446 -> [_ _ _ _ _ _ _ w484 _ _ _]
                          tunnel: w445 -> [_ _ _ _ _ _ _ _ w488 _ _]
                          tunnel: w444 -> [_ _ _ _ _ _ _ _ _ w492 _]
                          tunnel: [w454 w458 w462 w466 w470 w474 w478 w482 w486 w490 w494] -> w442
                          frame 0, Default {
                            n231 = property on="Frame Sync Edge for Channel 0" class="Enum (strict)"() -> ("Value"=w457:enum16{"Rising", "Falling"})  [unwired: 2 in, 2 out]
                            n232 = Equal?(x=w457, y=w456) -> (x = y?=w455:bool)
                            n233 = Not(x=w455) -> (.not. x?=w454:bool)
                          }
                          frame 1 {
                            n234 = property on="Channel Count Per Frame" class="DigNum (strict)"() -> ("Value"=w460:i32)  [unwired: 2 in, 2 out]
                            n235 = Equal?(x=w460, y=w461) -> (x = y?=w459:bool)
                            n236 = Not(x=w459) -> (.not. x?=w458:bool)
                          }
                          frame 2 {
                            n237 = property on="Channel Length" class="DigNum (strict)"() -> ("Value"=w464:i32)  [unwired: 2 in, 2 out]
                            n238 = Equal?(x=w465, y=w464) -> (x = y?=w463:bool)
                            n239 = Not(x=w463) -> (.not. x?=w462:bool)
                          }
                          frame 3 {
                            n240 = property on="Bit Depth" class="DigNum (strict)"() -> ("Value"=w468:i32)  [unwired: 2 in, 2 out]
                            n241 = Equal?(x=w469, y=w468) -> (x = y?=w467:bool)
                            n242 = Not(x=w467) -> (.not. x?=w466:bool)
                          }
                          frame 4 {
                            n243 = property on="Channel 0 Offset" class="DigNum (strict)"() -> ("Value"=w472:i32)  [unwired: 2 in, 2 out]
                            n244 = Equal?(x=w473, y=w472) -> (x = y?=w471:bool)
                            n245 = Not(x=w471) -> (.not. x?=w470:bool)
                          }
                          frame 5 {
                            n246 = property on="Endianness" class="Enum (strict)"() -> ("Value"=w476:enum16{"MSB First", "LSB First"})  [unwired: 2 in, 2 out]
                            n247 = Equal?(x=w477, y=w476) -> (x = y?=w475:bool)
                            n248 = Not(x=w475) -> (.not. x?=w474:bool)
                          }
                          frame 6 {
                            n249 = property on="Data Justification" class="Enum (strict)"() -> ("Value"=w480:enum16{"Left Justified", "Right Justified"})  [unwired: 2 in, 2 out]
                            n250 = Equal?(x=w481, y=w480) -> (x = y?=w479:bool)
                            n251 = Not(x=w479) -> (.not. x?=w478:bool)
                          }
                          frame 7 {
                            n252 = property on="Bit Clock Edge  Sync" class="Enum (strict)"() -> ("Value"=w485:enum16{"Rising", "Falling"})  [unwired: 2 in, 2 out]
                            n253 = Equal?(x=w484, y=w485) -> (x = y?=w483:bool)
                            n254 = Not(x=w483) -> (.not. x?=w482:bool)
                          }
                          frame 8 {
                            n255 = property on="Frame Length" class="DigNum (strict)"() -> ("Value"=w489:i32)  [unwired: 2 in, 2 out]
                            n256 = Equal?(x=w489, y=w488) -> (x = y?=w487:bool)
                            n257 = Not(x=w487) -> (.not. x?=w486:bool)
                          }
                          frame 9 {
                            n258 = property on="Frame Sync Pulse Width" class="DigNum (strict)"() -> ("Value"=w493:i32)  [unwired: 2 in, 2 out]
                            n259 = Equal?(x=w493, y=w492) -> (x = y?=w491:bool)
                            n260 = Not(x=w491) -> (.not. x?=w490:bool)
                          }
                          frame 10 {
                            w494 = TRUE
                          }
                        }
                      }
                      n261 = case shown="True" w428 {
                        tunnel: [TRUE ("T button?") w499] -> w429
                        frame True {
                        }
                        frame False {
                          n262 = Two Button Dialog(message="Do you want to save the changes in configurations?", 1:"Yes" ("F button name (\"Cancel\")"), 2:"No" ("T button name (\"OK\")")) -> (T button?=w499:bool)
                        }
                      }
                    }
                    frame Default {
                      n263 = Concatenate Strings("C:\\Users\\Public\\Documents\\National Instruments\\Audio\\Protocols\\" ("string"), w504) -> (w502:string)
                      n264 = String To Path(string=w502) -> (path=w501:path)
                      n265 = Open/Create/Replace File(file path (use dialog)=w501, operation (0:open)=T3."open") -> (refnum out=w521:refnum<file>)  [unwired: 4 in, 2 out]
                      n266 = Read from Text File(file (use dialog)=w521) -> (text=w522:string)  [unwired: 3 in, 3 out]
                      n267 = Unflatten From JSON(JSON string=w522, type and defaults=T2 {"Configurations"={"Frame_Sync_Edge_for_Channel 0"=1, "Channel_Count_Per_Frame"=2, "Channel_Length"=32, "Bit_Depth"=24, "Channel_0_Offset"=1, "Endianness"=0, "Data_Justification"=0, "Frame_Length"=64, "Frame_Sync_Pulse_Width"=32, "Bit_Clock_Edge_Sync"=0}}) -> (value=w520:T2)  [unwired: 5 in, 1 out]
                      n268 = Unbundle By Name(w520) -> ("Configurations"=w506:T4)
                      n269 = Unbundle By Name(w506) -> ("Frame_Sync_Edge_for_Channel 0"=w507:i32, "Channel_Count_Per_Frame"=w508:i32, "Channel_Length"=w509:i32, "Bit_Depth"=w510:i32, "Channel_0_Offset"=w511:i32, "Endianness"=w512:i32, "Data_Justification"=w513:i32, "Frame_Length"=w515:i32, "Frame_Sync_Pulse_Width"=w516:i32, "Bit_Clock_Edge_Sync"=w514:i32)
                      n270 = while {
                        tunnel: [w525] -> w517
                        tunnel: w516 -> [w535]
                        tunnel: w515 -> [w534]
                        tunnel: w514 -> [w533]
                        tunnel: w513 -> [w532]
                        tunnel: w512 -> [w531]
                        tunnel: w511 -> [w530]
                        tunnel: w510 -> [w529]
                        tunnel: w509 -> [w528]
                        tunnel: w508 -> [w527]
                        tunnel: w507 -> [w526]
                        i -> [w524]
                        stop <- w523 stop-if-true
                        n271 = case shown="0, Default" w524 {
                          tunnel: w526 -> [w536 _ _ _ _ _ _ _ _ _ _]
                          tunnel: [w538 w541 w545 w549 w553 w557 w561 w565 w569 w572 w576] -> w525
                          tunnel: w527 -> [_ w543 _ _ _ _ _ _ _ _ _]
                          tunnel: w528 -> [_ _ w547 _ _ _ _ _ _ _ _]
                          tunnel: w529 -> [_ _ _ w551 _ _ _ _ _ _ _]
                          tunnel: w530 -> [_ _ _ _ w555 _ _ _ _ _ _]
                          tunnel: w531 -> [_ _ _ _ _ w559 _ _ _ _ _]
                          tunnel: w532 -> [_ _ _ _ _ _ w563 _ _ _ _]
                          tunnel: w533 -> [_ _ _ _ _ _ _ w567 _ _ _]
                          tunnel: w534 -> [_ _ _ _ _ _ _ _ w571 _ _]
                          tunnel: w535 -> [_ _ _ _ _ _ _ _ _ w575 _]
                          tunnel: [w537 w540 w544 w548 w552 w556 w560 w564 w568 w573 w576] -> w523
                          frame 0, Default {
                            n272 = property on="Frame Sync Edge for Channel 0" class="Enum (strict)"() -> ("Value"=w539:enum16{"Rising", "Falling"})  [unwired: 2 in, 2 out]
                            n273 = Equal?(x=w539, y=w536) -> (x = y?=w538:bool)
                            n274 = Not(x=w538) -> (.not. x?=w537:bool)
                          }
                          frame 1 {
                            n275 = property on="Channel Count Per Frame" class="DigNum (strict)"() -> ("Value"=w542:i32)  [unwired: 2 in, 2 out]
                            n276 = Equal?(x=w542, y=w543) -> (x = y?=w541:bool)
                            n277 = Not(x=w541) -> (.not. x?=w540:bool)
                          }
                          frame 2 {
                            n278 = property on="Channel Length" class="DigNum (strict)"() -> ("Value"=w546:i32)  [unwired: 2 in, 2 out]
                            n279 = Equal?(x=w547, y=w546) -> (x = y?=w545:bool)
                            n280 = Not(x=w545) -> (.not. x?=w544:bool)
                          }
                          frame 3 {
                            n281 = property on="Bit Depth" class="DigNum (strict)"() -> ("Value"=w550:i32)  [unwired: 2 in, 2 out]
                            n282 = Equal?(x=w551, y=w550) -> (x = y?=w549:bool)
                            n283 = Not(x=w549) -> (.not. x?=w548:bool)
                          }
                          frame 4 {
                            n284 = property on="Channel 0 Offset" class="DigNum (strict)"() -> ("Value"=w554:i32)  [unwired: 2 in, 2 out]
                            n285 = Equal?(x=w555, y=w554) -> (x = y?=w553:bool)
                            n286 = Not(x=w553) -> (.not. x?=w552:bool)
                          }
                          frame 5 {
                            n287 = property on="Endianness" class="Enum (strict)"() -> ("Value"=w558:enum16{"MSB First", "LSB First"})  [unwired: 2 in, 2 out]
                            n288 = Equal?(x=w559, y=w558) -> (x = y?=w557:bool)
                            n289 = Not(x=w557) -> (.not. x?=w556:bool)
                          }
                          frame 6 {
                            n290 = property on="Data Justification" class="Enum (strict)"() -> ("Value"=w562:enum16{"Left Justified", "Right Justified"})  [unwired: 2 in, 2 out]
                            n291 = Equal?(x=w563, y=w562) -> (x = y?=w561:bool)
                            n292 = Not(x=w561) -> (.not. x?=w560:bool)
                          }
                          frame 7 {
                            n293 = property on="Bit Clock Edge  Sync" class="Enum (strict)"() -> ("Value"=w566:enum16{"Rising", "Falling"})  [unwired: 2 in, 2 out]
                            n294 = Equal?(x=w567, y=w566) -> (x = y?=w565:bool)
                            n295 = Not(x=w565) -> (.not. x?=w564:bool)
                          }
                          frame 8 {
                            n296 = property on="Frame Length" class="DigNum (strict)"() -> ("Value"=w570:i32)  [unwired: 2 in, 2 out]
                            n297 = Equal?(x=w570, y=w571) -> (x = y?=w569:bool)
                            n298 = Not(x=w569) -> (.not. x?=w568:bool)
                          }
                          frame 9 {
                            n299 = property on="Frame Sync Pulse Width" class="DigNum (strict)"() -> ("Value"=w574:i32)  [unwired: 2 in, 2 out]
                            n300 = Equal?(x=w574, y=w575) -> (x = y?=w572:bool)
                            n301 = Not(x=w572) -> (.not. x?=w573:bool)
                          }
                          frame 10 {
                            w576 = TRUE
                          }
                        }
                      }
                      n302 = case shown="False" w517 {
                        tunnel: [TRUE ("T button?") w581] -> w505
                        frame True {
                        }
                        frame False {
                          n303 = Two Button Dialog(message="Do you want to save changes in file?", 1:"Yes" ("F button name (\"Cancel\")"), 2:"No" ("T button name (\"OK\")")) -> (T button?=w581:bool)
                        }
                      }
                    }
                  }
                }
              }
            }
          }
        }
      }
    }
  }
  n304 = control-ref of="This VI"() -> (w22:refnum<vi>)
  n305 = invoke class="VI" method="FP.Close"(reference=w22, error in=w21) -> (error out=→"error out":errorcluster)  [unwired: 1 in, 2 out]
